vi "AK Befehl Auswerten - PEUS.vi"(10 "Array":string[](array[string])) -> (2 "String für schreiben":string)   [LabVIEW 2020, in "AK-Schnittstelle.lvlib"]
uses:
  AK-Schnittstelle.lvlib
  Aktionen Stoernummern pruefen.ctl
  Aktionen Zustandsfehlerinformation.ctl
  Aktionen Gespeicherte Werte.ctl
  Funktionstasten/Zustaende.ctl
  Funktionstasten/Funktionstasten-Aktion.ctl
  Funktionstasten/Betriebsart.ctl
  Seiten/Log Konfig/Aktionen Trigger.ctl
  Seiten/Erweiterte Konfig/FGV PID Aktionen.ctl
  Seiten/FT-IR/FGV FT-IR Diagnose Aktionen.ctl
  AK Namen Aktionen.ctl
  Seiten/System Einstellungen V2/Aktioen FGV System.ctl
  Messdaten/Aktionen FGV Messdaten.ctl
  Schedule Modul/Aktion FGV Scheduler Status.ctl
  Funktionstasten/Funktionstasten.lvlib
  Seiten/Log Konfig/LogKonfig.lvlib
  Seiten/FT-IR/FT-IR.lvlib
  Seiten/FT-IR/FGV FT-IR Gasliste Aktionen.ctl
  Messdaten/Messdaten.lvlib
  Seiten/Erweiterte Konfig/Erweiterte Konfig.lvlib
  cRIO/PC/Kommunikation mit cRIO.lvlib
  Seiten/System Einstellungen V2/System Einstellungen V2.lvlib
  Schedule Modul/Schedule Modul.lvlib
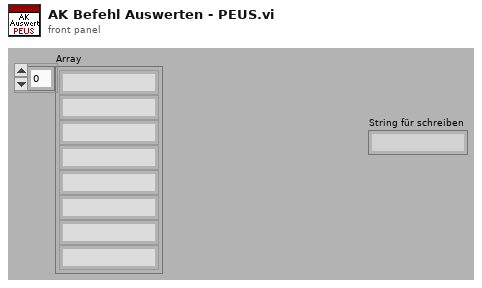
[diagram p1: front panel]
types:
  T1 = typedef "AK-Schnittstelle.lvlib/Aktionen Stoernummern pruefen.ctl" = enum16{"lesen", "prüfen"}
  T2 = typedef "AK-Schnittstelle.lvlib/Aktionen Zustandsfehlerinformation.ctl" = enum16{"OK", "Offline", "Busy", "Syntax Error", "Datenfehler"}
  T3 = typedef "AK-Schnittstelle.lvlib/Aktionen Gespeicherte Werte.ctl" = enum16{"lesen", "laden", "speichern", "Seriell", "TCP", "Diverse", "AKTIV", "AK-Namen"}
  T4 = typedef "Funktionstasten.lvlib/Zustaende.ctl" = enum16{"Standby", "Pause", "Eco", "Messen", "Kalibrieren", "Spülen Filter", "Spülen Leitung", "Umgebungsluft", "0-Gas", "Cal-Gas", "CG zu PNS", "-------------", "Init 1", "Init 2", "Init 3", "Init 4", "Messen vorbereiten", "Messen durchführen", "Exit"}
  T5 = typedef "Funktionstasten.lvlib/Betriebsart.ctl" = enum16{"Manuell", "Remote", "Bitparallel"}
  T6 = typedef "Funktionstasten.lvlib/Funktionstasten-Aktion.ctl" = enum16{"Initialisieren", "Zustand setzen", "Taste gedrückt", "Fehler speichern", "Lesen", "Manuell", "Remote", "Bitparallel", "Samplepoint", "Zeit Prüfen", "reset Umschalten"}
  T7 = typedef "LogKonfig.lvlib/Aktionen Trigger.ctl" = enum16{"lesen", "ALLE schreiben", "Trigger prüfen", "Trigger rücksetzen"}
  T8 = typedef "Erweiterte Konfig.lvlib/FGV PID Aktionen.ctl" = enum16{"Lesen", "Schreiben PID", "Schreiben Sonstige", "Dichtheitstest", "Aktionen Dicht.", "Parameter Sensor"}
  T9 = typedef "FT-IR.lvlib/FGV FT-IR Diagnose Aktionen.ctl" = enum16{"Lesen", "Diagnose Schreiben", "Min Schreiben", "Max Schreiben"}
  T10 = typedef "AK-Schnittstelle.lvlib/AK Namen Aktionen.ctl" = enum16{"lesen", "laden", "speichern Namen", "AK Namen", "Liste erstellen", "EKFG erstellen", "speichern EKFG", "EKFG schreiben", "Neuen Eintrag erzeugen"}
  T11 = typedef "FT-IR.lvlib/FGV FT-IR Gasliste Aktionen.ctl" = enum16{"lesen", "Gasliste FT-IR", "Gasliste ausgelesen", "laden", "speichern", "löschen"}
  T12 = typedef "System Einstellungen V2.lvlib/Aktioen FGV System.ctl" = enum16{"lesen", "laden", "speichern", "Optionen schreiben", "Zeitstempel", "Reset BMP", "Reset SQP", "Wartung", "Werkseinstellung"}
  T13 = typedef "Messdaten.lvlib/Aktionen FGV Messdaten.ctl" = enum16{"lesen", "schreiben", "löschen", "Mittelwerte", "Komponente"}
  T14 = typedef "Schedule Modul.lvlib/Aktion FGV Scheduler Status.ctl" = enum16{"lesen", "init", "aktiv", "inaktiv"}
  T15 = typedef "AK-Schnittstelle.lvlib/Diverse gespeicherte Werte.ctl" = cluster{"Kalibriergaseingang":i16, "SamplePoint":i16, "CalGas zu PNS":i16, "Gas-Reihenfolge":i16[], "Zeit 0-Gas":sgl, "Zeit CalGas":sgl, "AK Befehlssatz":T16}
  T16 = typedef "AK-Schnittstelle.lvlib/AK Befehlssatz.ctl" = enum16{"MEXA", "IAG v1.4", "AVL (Puma)", "PEUS"}
  T17 = typedef "LogKonfig.lvlib/Element Triggerereignisse.ctl" = cluster{"Trigger verwenden":T18, "Messwert":u16, "kl./gr.":u16, "Wert":sgl, "Puffergröße":sgl}
  T18 = typedef "LogKonfig.lvlib/Auswahlfeld aktiviert-deaktiviert.ctl" = u16
  T19 = typedef "Verwaltung - cRIO.lvlib/Analog Eingaenge.ctl" = cluster{"AI0: Durchfluss FT-IR":sgl, "AI1: Druck Ausgang":sgl, "AI2: Umgebungsdruck":sgl, "AI3: Druck FT-IR":sgl, "AI4: Druck CalGas":sgl, "AI5: Reserve":sgl, "AI6: Reserve":sgl, "AI7: Reserve":sgl, "Rohwert Durchfluss FT-IR":sgl, "Rohwert Druck Ausgang":sgl, "Rohwert Umgebungsdruck":sgl, "Rohwert Druck FT-IR":sgl, "Rohwert Druck CalGas":sgl, "Rohwert AI5":sgl, "Rohwert AI6":sgl, "Rohwert AI7":sgl, "Rohwert Diffdruck mbar FTIR":sgl}
  T20 = typedef "System Einstellungen V2.lvlib/Optionen.ctl" = cluster{"Störmeldep.":bool, "Betriebszustände":bool, "AK in ppm":bool, "log Cal-Gas":bool, "log 0-Gas":bool, "Durchflusssensor 0-5V":bool, "PNS?":bool, "Mit N2 spülen":bool, "TRE08":bool, "Amium 10-Fach":bool, "Verticale Scrollbar aktiv":bool, "Loggingtakt":bool, "AK Rezeptwechsel gleich wie MKS":bool, "NG ECO":bool}
  T21 = typedef "Verwaltung - cRIO.lvlib/TC Eingaenge.ctl" = cluster{"TC0: Reserve":sgl, "TC1: HL zu FT-IR":sgl, "TC2: HL Extern SP1":sgl, "TC3: HL Extern SP2":sgl, "TC4: Reserve":sgl, "TC5: Reserve":sgl, "TC6: Reserve":sgl, "TC7: Reserve":sgl, "TC8: FT-IR":sgl, "TC9: Reserve":sgl, "TC10: Schaltschrank":sgl, "TC11: Umgebung":sgl}
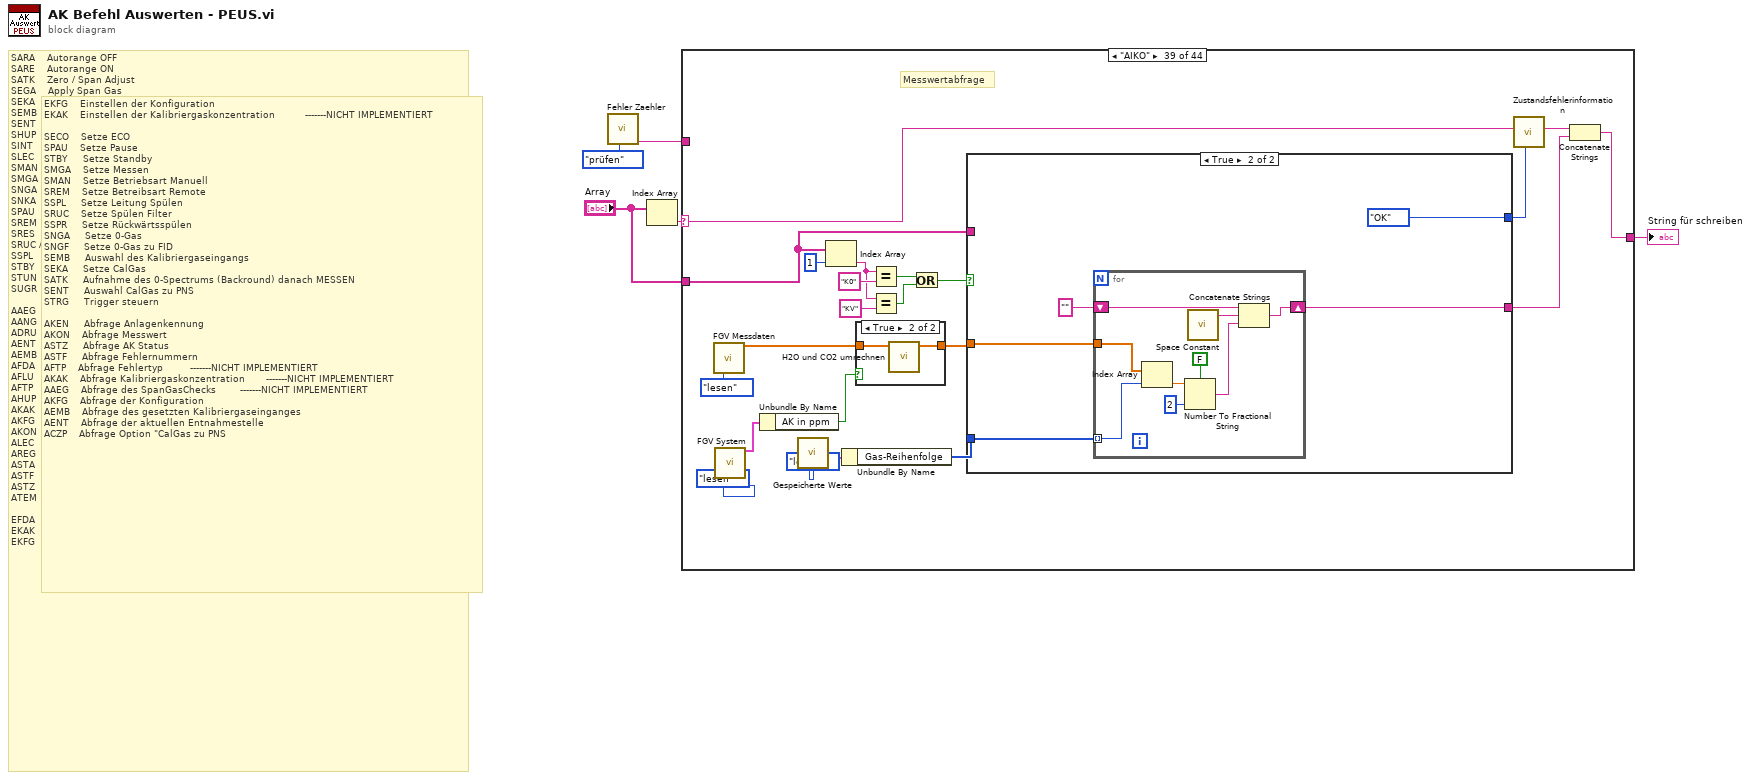
[diagram p0: block diagram]
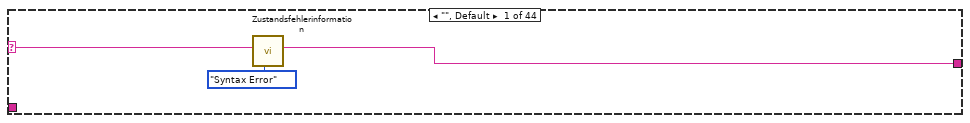
[diagram p2: hidden frame]
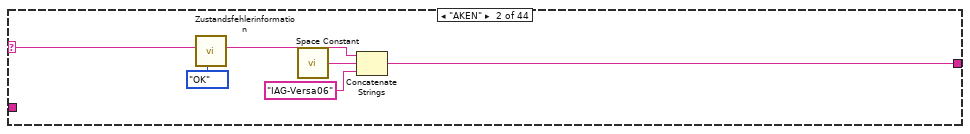
[diagram p3: hidden frame]
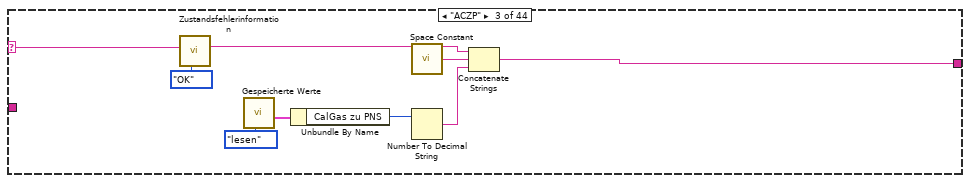
[diagram p4: hidden frame]
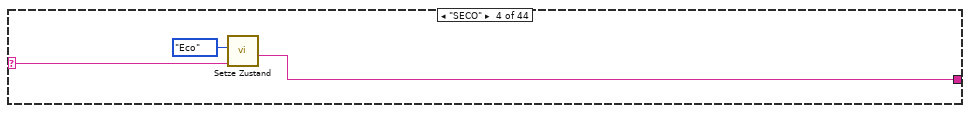
[diagram p5: hidden frame]
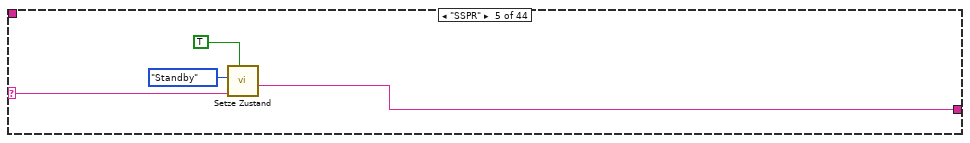
[diagram p6: hidden frame]
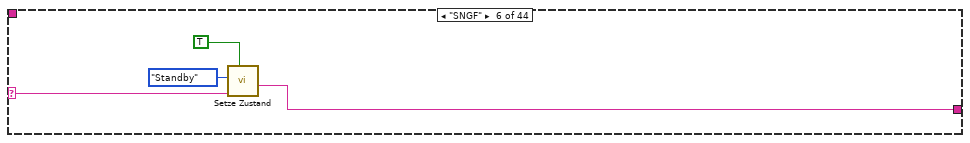
[diagram p7: hidden frame]
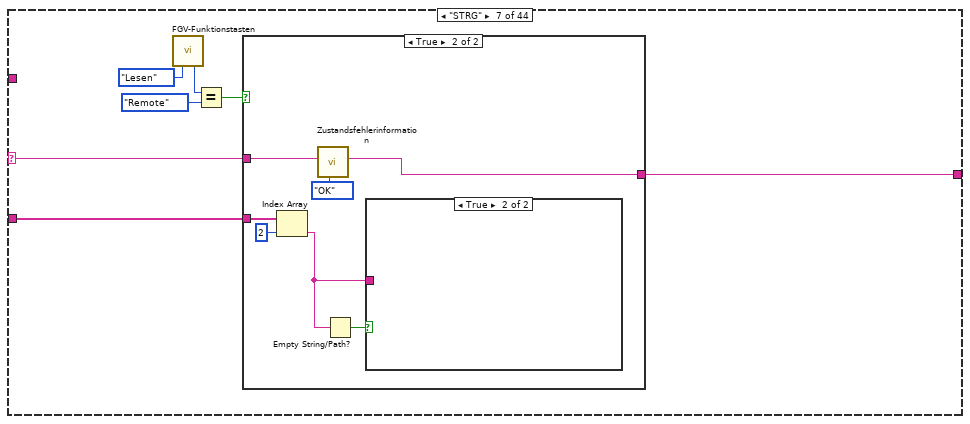
[diagram p8: hidden frame]
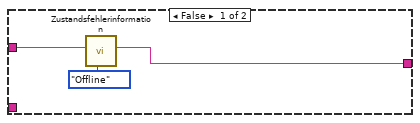
[diagram p9: hidden frame]
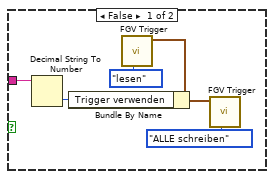
[diagram p10: hidden frame]
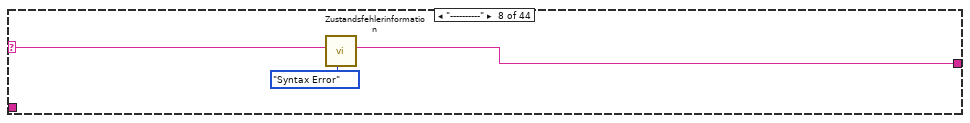
[diagram p11: hidden frame]
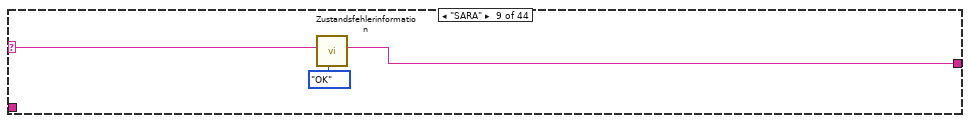
[diagram p12: hidden frame]
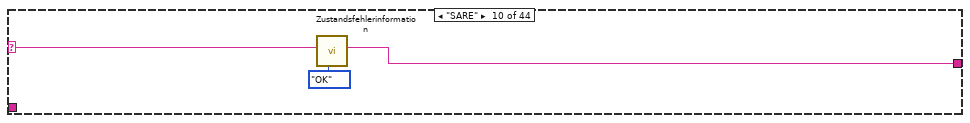
[diagram p13: hidden frame]
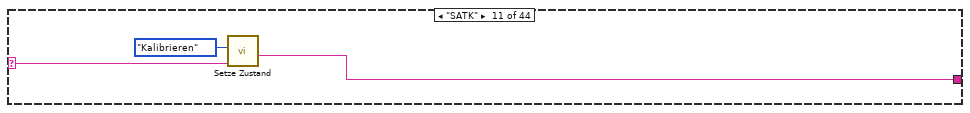
[diagram p14: hidden frame]
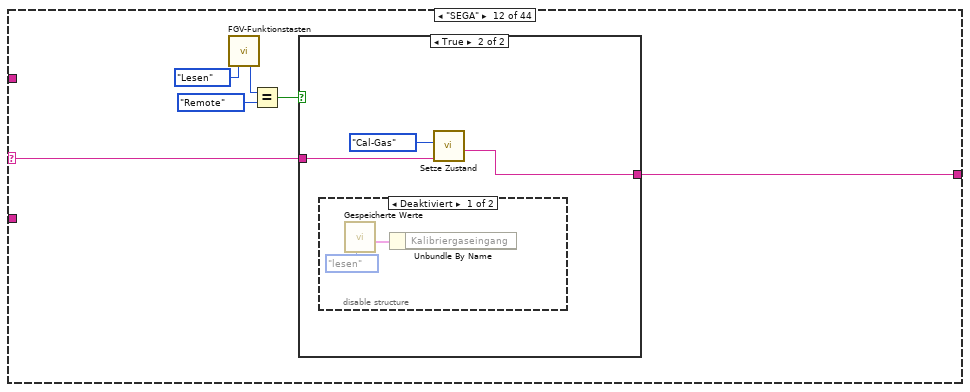
[diagram p15: hidden frame]
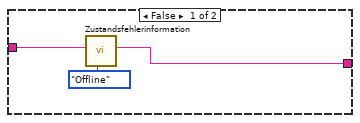
[diagram p16: hidden frame]
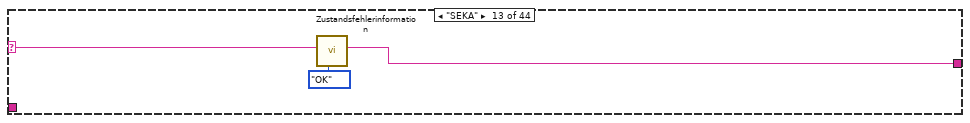
[diagram p18: hidden frame]
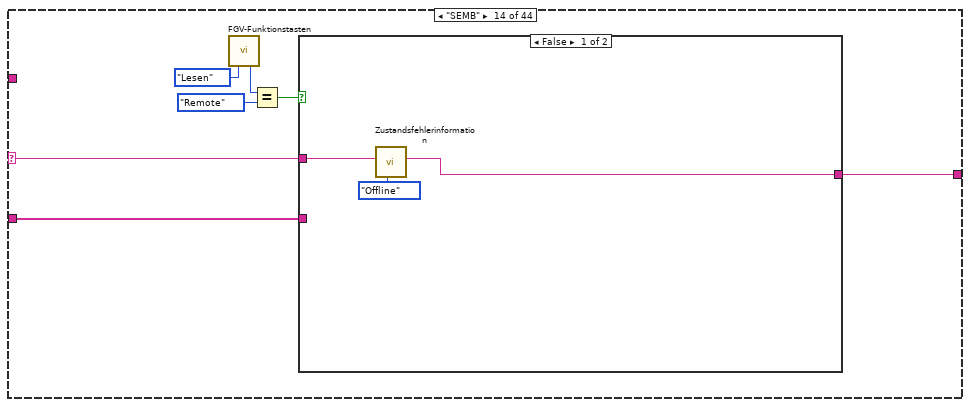
[diagram p19: hidden frame]
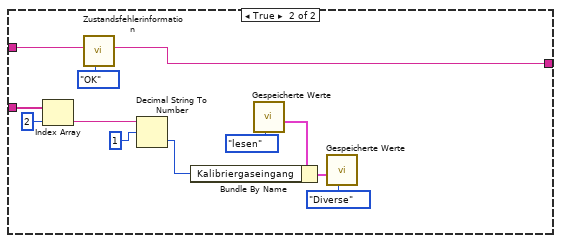
[diagram p20: hidden frame]
diagram:
  # "SARA    Autorange OFF\nSARE    Autorange ON\nSATK    Zero / Span Adjust\nSEGA    Apply Span Gas\nSEKA    Performing FTIR Span Gas Check\nSEMB    Selecting Calibration Gas Inlet\nSENT    Set Sampling\nSHUP    Hang-Up Test         -------NICHT IMPLEMENTIERT\nSINT     Starting Continous FTIR Measurement\nSLEC     Leak Check\nSMAN    Set Manual\nSMGA    Set Measure\nSNGA    Apply Zero Gas\nSNKA    Adjust Zero Point\nSPAU    Pause Modus\nSREM    Set Remote\nSRES    Set Reset\nSRUC / SRUK  Backflush\nSSPL     Purge Gas Lines\nSTBY    Set Standby\nSTUN    Automatically Adjusting Optics and Signals         -------NICHT IMPLEMENTIERT\nSUGR    Recording Zero Energy Spectrum\n\nAAEG    Inquire Span Point Deviation\nAANG    Inquire Zero Point Deviation\nADRU    Inquire Pressure of SESAM FTIR\nAENT    Inquire Sampling Points\nAEMB    Inquire Measuring Range\nAFDA    Inquire Function Duration\nAFLU     Inquire Sample Flow of SBEAM FTIR\nAFTP     Inquire Error Type\nAHUP    Inquire Hangup Result         -------NICHT IMPLEMENTIERT\nAKAK    Inquire Span Gas Concentrations         -------NICHT IMPLEMENTIERT\nAKFG    Inquire Configuration\nAKON   Inquire Measuring Value\nALEC    Inquire Leak Check Result         -------NICHT IMPLEMENTIERT\nAREG    Inquire Control Variable of SESAM FTIR          -------NICHT IMPLEMENTIERT\nASTA    Inquire Erroneous Channel         -------NICHT IMPLEMENTIERT\nASTF    Inquire Error Numbers\nASTZ    Inquire AK Status\nATEM   Inquire Temperature of SESAM FTIR\n\nEFDA   Configure Function Duration\nEKAK   Configure Span Gas Concentration         -------NICHT IMPLEMENTIERT\nEKFG   Configure Configuration"
  # "EKFG    Einstellen der Konfiguration\nEKAK    Einstellen der Kalibriergaskonzentration          -------NICHT IMPLEMENTIERT\n\nSECO    Setze ECO\nSPAU    Setze Pause\nSTBY     Setze Standby\nSMGA    Setze Messen\nSMAN    Setze Betriebsart Manuell\nSREM    Setze Betreibsart Remote\nSSPL     Setze Leitung Spülen\nSRUC    Setze Spülen Filter\nSSPR     Setze Rückwärtsspülen\nSNGA     Setze 0-Gas\nSNGF     Setze 0-Gas zu FID\nSEMB     Auswahl des Kalibriergaseingangs\nSEKA     Setze CalGas\nSATK     Aufnahme des 0-Spectrums (Backround) danach MESSEN\nSENT     Auswahl CalGas zu PNS\nSTRG     Trigger steuern\n\nAKEN     Abfrage Anlagenkennung\nAKON    Abfrage Messwert\nASTZ     Abfrage AK Status\nASTF     Abfrage Fehlernummern\nAFTP    Abfrage Fehlertyp         -------NICHT IMPLEMENTIERT\nAKAK    Abfrage Kalibriergaskonzentration       -------NICHT IMPLEMENTIERT\nAAEG    Abfrage des SpanGasChecks        -------NICHT IMPLEMENTIERT\nAKFG    Abfrage der Konfiguration\nAEMB    Abfrage des gesetzten Kalibriergaseinganges\nAENT    Abfrage der aktuellen Entnahmestelle\nACZP    Abfrage Option \"CalGas zu PNS"
  n1 = call "Fehler Zaehler.vi"("Aktionen"=Aktionen_Stoernummern_pruefen."prüfen") -> ("Fehlerzähler"=w3:string)  [unwired: 7 in, 3 out]
  n2 = Index Array(array="Array") -> (element=w2:string)  [unwired: 1 in]
  n3 = case shown="\"AIKO\"" w2 {
    selector: w2 -> [w7 w11 w21 w26 w30 w34 w37 w59 w62 w65 w68 w71 w85 w89 w112 w149 w152 w162 w176 w179 w181 w185 w187 w191 w195 w198 w201 w204 w206 w220 w228 w244 w250 w256 w287 w297 w305 w365 w439 w493 w511 w563 w572 w600]
    tunnel: [w6 w13 w23 w25 w29 w33 w36 w58 w61 w64 w67 w70 w84 w88 w111 w148 w151 w161 w175 w178 w180 w184 w186 w190 w194 w197 w200 w203 w205 w222 w230 w246 w252 w257 w289 w299 w307 w366 w440 w495 w509 w565 w571 w599] -> w5
    tunnel: w3 -> [_ _ _ _ _ _ _ _ _ _ _ _ _ _ _ _ _ _ _ _ _ _ _ _ _ _ _ _ _ _ _ _ _ _ _ _ _ _ _ _ _ _ _ _]
    tunnel: "Array" -> [_ _ _ _ _ _ w35 _ _ _ _ _ _ w87 w110 _ _ _ _ _ _ _ _ _ _ _ _ _ _ _ _ _ _ w255 _ _ w302 w359 w433 _ w510 _ w570 w601]
    frame "", Default {
      n4 = call "Zustandsfehlerinformation.vi"("Aktionen"=Aktionen_Zustandsfehlerinformation."Syntax Error", "String"=w7) -> ("String"=w6:string)  [unwired: 9 in]
    }
    frame "AKEN" {
      n5 = call "Zustandsfehlerinformation.vi"("Aktionen"=Aktionen_Zustandsfehlerinformation."OK", "String"=w11) -> ("String"=w10:string)  [unwired: 9 in]
      n6 = call <vilib>:"Space Constant.vi"() -> ("String"=w9:string)
      n7 = Concatenate Strings(w10, w9, "IAG-Versa06" ("String")) -> (w13:string)
    }
    frame "ACZP" {
      n8 = call "Zustandsfehlerinformation.vi"("Aktionen"=Aktionen_Zustandsfehlerinformation."OK", "String"=w21) -> ("String"=w20:string)  [unwired: 9 in]
      n9 = call "Gespeicherte Werte.vi"("Aktionen"=Aktionen_Gespeicherte_Werte."lesen") -> ("Diverse Werte"=w15:T15)  [unwired: 6 in, 4 out]
      n10 = Unbundle By Name(w15) -> ("CalGas zu PNS"=w18:i16)
      n11 = call <vilib>:"Space Constant.vi"() -> ("String"=w16:string)
      n12 = Number To Decimal String(number=w18) -> (decimal integer string=w17:string)  [unwired: 1 in]
      n13 = Concatenate Strings(w20, w16, w17) -> (w23:string)
    }
    frame "SECO" {
      n14 = call "Setze Zustand.vi"("AK Befehl"=w26, "Zustand"=Zustaende."Eco") -> ("Antwort String"=w25:string)  [unwired: 8 in, 1 out]
    }
    frame "SSPR" {
      n15 = call "Setze Zustand.vi"("Befehl nicht vorhanden!"=TRUE, "AK Befehl"=w30, "Zustand"=Zustaende."Standby") -> ("Antwort String"=w29:string)  [unwired: 7 in, 1 out]
    }
    frame "SNGF" {
      n16 = call "Setze Zustand.vi"("Befehl nicht vorhanden!"=TRUE, "AK Befehl"=w34, "Zustand"=Zustaende."Standby") -> ("Antwort String"=w33:string)  [unwired: 7 in, 1 out]
    }
    frame "STRG" {
      n17 = call "FGV-Funktionstasten.vi"("Aktion"=Funktionstasten-Aktion."Lesen") -> ("Betriebsart"=w40:T5)  [unwired: 7 in, 7 out]
      n18 = Equal?(x=w40, y=Betriebsart."Remote" ("Betriebsart")) -> (x = y?=w41:bool)
      n19 = case shown="True" w41 {
        tunnel: w37 -> [w43 w50]
        tunnel: [w42 w49] -> w36
        tunnel: w35 -> [_ w48]
        frame False {
          n20 = call "Zustandsfehlerinformation.vi"("Aktionen"=Aktionen_Zustandsfehlerinformation."Offline", "String"=w43) -> ("String"=w42:string)  [unwired: 9 in]
        }
        frame True {
          n21 = Index Array(array=w48, index=2 ("Index")) -> (element=w46:string)
          n22 = call "Zustandsfehlerinformation.vi"("Aktionen"=Aktionen_Zustandsfehlerinformation."OK", "String"=w50) -> ("String"=w49:string)  [unwired: 9 in]
          n23 = Empty String/Path?(string/path=w46) -> (empty?=w45:bool)
          n24 = case shown="True" w45 {
            tunnel: w46 -> [w57 _]
            frame False {
              n25 = Decimal String To Number(string=w57) -> (number=w54:i32)  [unwired: 2 in, 1 out]
              n26 = call "FGV Trigger.vi"("Aktion"=Aktionen_Trigger."lesen") -> ("Triggerereignis neu"=w53:T17)  [unwired: 7 in, 3 out]
              n27 = Bundle By Name(cluster=w53, "Trigger verwenden"=w54) -> (w52:T17)
              n28 = call "FGV Trigger.vi"("Aktion"=Aktionen_Trigger."ALLE schreiben", "Triggerereignis"=w52) -> ()  [unwired: 6 in, 4 out]
            }
            frame True {
            }
          }
        }
      }
    }
    frame "----------" {
      n29 = call "Zustandsfehlerinformation.vi"("Aktionen"=Aktionen_Zustandsfehlerinformation."Syntax Error", "String"=w59) -> ("String"=w58:string)  [unwired: 9 in]
    }
    frame "SARA" {
      n30 = call "Zustandsfehlerinformation.vi"("Aktionen"=Aktionen_Zustandsfehlerinformation."OK", "String"=w62) -> ("String"=w61:string)  [unwired: 9 in]
    }
    frame "SARE" {
      n31 = call "Zustandsfehlerinformation.vi"("Aktionen"=Aktionen_Zustandsfehlerinformation."OK", "String"=w65) -> ("String"=w64:string)  [unwired: 9 in]
    }
    frame "SATK" {
      n32 = call "Setze Zustand.vi"("AK Befehl"=w68, "Zustand"=Zustaende."Kalibrieren") -> ("Antwort String"=w67:string)  [unwired: 8 in, 1 out]
    }
    frame "SEGA" {
      n33 = call "FGV-Funktionstasten.vi"("Aktion"=Funktionstasten-Aktion."Lesen") -> ("Betriebsart"=w74:T5)  [unwired: 7 in, 7 out]
      n34 = Equal?(x=w74, y=Betriebsart."Remote" ("Betriebsart")) -> (x = y?=w75:bool)
      n35 = case shown="True" w75 {
        tunnel: w71 -> [w77 w80]
        tunnel: [w76 w79] -> w70
        frame False {
          n36 = call "Zustandsfehlerinformation.vi"("Aktionen"=Aktionen_Zustandsfehlerinformation."Offline", "String"=w77) -> ("String"=w76:string)  [unwired: 9 in]
        }
        frame True {
          n37 = disable-structure shown="Deaktiviert" {
            frame Disabled {
              n38 = call "Gespeicherte Werte.vi"("Aktionen"=Aktionen_Gespeicherte_Werte."lesen") -> ("Diverse Werte"=w82:T15)  [unwired: 6 in, 4 out]
              n39 = Unbundle By Name(w82) -> ()  [unwired: 1 out]
            }
            frame Enabled {
            }
          }
          n40 = call "Setze Zustand.vi"("AK Befehl"=w80, "Zustand"=Zustaende."Cal-Gas") -> ("Antwort String"=w79:string)  [unwired: 8 in, 1 out]
        }
      }
    }
    frame "SEKA" {
      n41 = call "Zustandsfehlerinformation.vi"("Aktionen"=Aktionen_Zustandsfehlerinformation."OK", "String"=w85) -> ("String"=w84:string)  [unwired: 9 in]
    }
    frame "SEMB" {
      n42 = call "FGV-Funktionstasten.vi"("Aktion"=Funktionstasten-Aktion."Lesen") -> ("Betriebsart"=w92:T5)  [unwired: 7 in, 7 out]
      n43 = Equal?(x=w92, y=Betriebsart."Remote" ("Betriebsart")) -> (x = y?=w93:bool)
      n44 = case shown="False" w93 {
        tunnel: w89 -> [w95 w107]
        tunnel: [w94 w106] -> w88
        tunnel: w87 -> [_ w105]
        frame False {
          n45 = call "Zustandsfehlerinformation.vi"("Aktionen"=Aktionen_Zustandsfehlerinformation."Offline", "String"=w95) -> ("String"=w94:string)  [unwired: 9 in]
        }
        frame True {
          n46 = Index Array(array=w105, index=2 ("Index")) -> (element=w98:string)
          n47 = call "Zustandsfehlerinformation.vi"("Aktionen"=Aktionen_Zustandsfehlerinformation."OK", "String"=w107) -> ("String"=w106:string)  [unwired: 9 in]
          n48 = Decimal String To Number(string=w98, offset=1 ("Offset (0)")) -> (number=w97:i32)  [unwired: 1 in, 1 out]
          n49 = call "Gespeicherte Werte.vi"("Aktionen"=Aktionen_Gespeicherte_Werte."lesen") -> ("Diverse Werte"=w100:T15)  [unwired: 6 in, 4 out]
          n50 = Bundle By Name(cluster=w100, "Kalibriergaseingang"=w97) -> (w99:T15)
          n51 = call "Gespeicherte Werte.vi"("Aktionen"=Aktionen_Gespeicherte_Werte."Diverse", "Diverse Werte"=w99) -> ()  [unwired: 5 in, 5 out]
        }
      }
    }
    frame "SENT" {
      n52 = call "FGV-Funktionstasten.vi"("Aktion"=Funktionstasten-Aktion."Lesen") -> ("Betriebsart"=w115:T5)  [unwired: 7 in, 7 out]
      n53 = Equal?(x=w115, y=Betriebsart."Remote" ("Betriebsart")) -> (x = y?=w109:bool)
      n54 = case shown="True" w109 {
        tunnel: w112 -> [w117 w131]
        tunnel: [w116 w130] -> w111
        tunnel: w110 -> [_ w120]
        frame False {
          n55 = call "Zustandsfehlerinformation.vi"("Aktionen"=Aktionen_Zustandsfehlerinformation."Offline", "String"=w117) -> ("String"=w116:string)  [unwired: 9 in]
        }
        frame True {
          n56 = Index Array(array=w120, index=2 ("Index")) -> (element=w122:string)
          n57 = Equal?(x=w122, y="L1") -> (x = y?=w119:bool)
          n58 = case shown="True" w119 {
            tunnel: [w142 w143] -> w124
            tunnel: w120 -> [w133 w145]
            frame False {
              n59 = Array Size(array=w133) -> (size(s)=w140:i32)
              n60 = Greater?(x=w140, y=3) -> (0:w138:bool)
              n61 = Select(t=3, s=w138, f=2 ("Index")) -> (s? t:f=w135:i32)
              n62 = Index Array(array=w133, index=w135) -> (element=w134:string)
              n63 = Decimal String To Number(string=w134, offset=1 ("Offset")) -> (number=w142:i32)  [unwired: 1 in, 1 out]
            }
            frame True {
              n64 = Index Array(array=w145, index=3 ("Index")) -> (element=w144:string)
              n65 = Decimal String To Number(string=w144) -> (number=w143:i32)  [unwired: 2 in, 1 out]
            }
          }
          n66 = call "FGV-Funktionstasten.vi"("Samplepoint"=w124, "Aktion"=Funktionstasten-Aktion."Samplepoint") -> ()  [unwired: 6 in, 8 out]
          n67 = call "Zustandsfehlerinformation.vi"("Aktionen"=Aktionen_Zustandsfehlerinformation."OK", "String"=w131) -> ("String"=w130:string)  [unwired: 9 in]
          n68 = call "Gespeicherte Werte.vi"("Aktionen"=Aktionen_Gespeicherte_Werte."lesen") -> ("Diverse Werte"=w127:T15)  [unwired: 6 in, 4 out]
          n69 = Bundle By Name(cluster=w127, "SamplePoint"=w124) -> (w126:T15)
          n70 = call "Gespeicherte Werte.vi"("Aktionen"=Aktionen_Gespeicherte_Werte."Diverse", "Diverse Werte"=w126) -> ()  [unwired: 5 in, 5 out]
        }
      }
    }
    frame "SINT" {
      n71 = call "Setze Zustand.vi"("AK Befehl"=w149, "Zustand"=Zustaende."Messen") -> ("Antwort String"=w148:string)  [unwired: 8 in, 1 out]
    }
    frame "SLEC" {
      n72 = flat-sequence {
        frame #0 {
          n73 = call "FGV Erweiterte Konfig.vi"("Aktion"=FGV_PID_Aktionen."Dichtheitstest", "Dichtheitstest?"=TRUE) -> ()  [unwired: 5 in, 5 out]
        }
        frame #1 {
          n74 = vi-ref "Dichtheitstest.vi"() -> (w157:refnum<vi>)
          n75 = invoke class="VI" method="VI ausführen"(reference=w157, "Wait until done"=FALSE ("Warten bis beendet"), "Auto Dispose Ref"=TRUE ("Referenz automatisch schließen")) -> (reference out=w158:refnum<vi>, error out=w156:errorcluster)  [unwired: 2 in, 3 out]
          n76 = invoke class="VI" method="FP.Öffnen"(reference=w158, error in=w156) -> (error out=w155:errorcluster)  [unwired: 3 in, 4 out]
          n77 = call <vilib>:"Clear Errors.vi"("error in (no error)"=w155) -> ()  [unwired: 5 in, 2 out]
        }
      }
      n78 = call "Setze Zustand.vi"("AK Befehl"=w152, "Zustand"=Zustaende."Standby") -> ("Antwort String"=w151:string)  [unwired: 8 in, 1 out]
    }
    frame "SMAN" {
      n79 = call "FGV-Funktionstasten.vi"("Aktion"=Funktionstasten-Aktion."Lesen") -> ("Betriebsart"=w166:T5)  [unwired: 7 in, 7 out]
      n80 = Equal?(x=w166, y=Betriebsart."Remote" ("Betriebsart")) -> (x = y?=w163:bool)
      n81 = case shown="True" w163 {
        tunnel: w162 -> [w169 w172]
        tunnel: [w167 w171] -> w161
        frame False {
          n82 = call "Zustandsfehlerinformation.vi"("Aktionen"=Aktionen_Zustandsfehlerinformation."Offline", "String"=w169) -> ("String"=w167:string)  [unwired: 9 in]
        }
        frame True {
          n83 = call "Zustandsfehlerinformation.vi"("Aktionen"=Aktionen_Zustandsfehlerinformation."OK", "String"=w172) -> ("String"=w171:string)  [unwired: 9 in]
          n84 = call "FGV-Funktionstasten.vi"("Aktion"=Funktionstasten-Aktion."Manuell") -> ()  [unwired: 7 in, 8 out]
        }
      }
    }
    frame "SMGA" {
      n85 = call "Setze Zustand.vi"("AK Befehl"=w176, "Zustand"=Zustaende."Messen") -> ("Antwort String"=w175:string)  [unwired: 8 in, 1 out]
    }
    frame "SNGA" {
      n86 = call "Setze Zustand.vi"("AK Befehl"=w179, "Zustand"=Zustaende."0-Gas") -> ("Antwort String"=w178:string)  [unwired: 8 in, 1 out]
    }
    frame "SNKA" {
      n87 = call "Zustandsfehlerinformation.vi"("Aktionen"=Aktionen_Zustandsfehlerinformation."OK", "String"=w181) -> ("String"=w180:string)  [unwired: 9 in]
    }
    frame "SPAU" {
      n88 = call "Setze Zustand.vi"("AK Befehl"=w185, "Zustand"=Zustaende."Pause") -> ("Antwort String"=w184:string)  [unwired: 8 in, 1 out]
    }
    frame "SREM" {
      n89 = call "Zustandsfehlerinformation.vi"("Aktionen"=Aktionen_Zustandsfehlerinformation."OK", "String"=w187) -> ("String"=w186:string)  [unwired: 9 in]
      n90 = call "FGV-Funktionstasten.vi"("Aktion"=Funktionstasten-Aktion."Remote") -> ()  [unwired: 7 in, 8 out]
    }
    frame "SRES" {
      n91 = call "Zustandsfehlerinformation.vi"("Aktionen"=Aktionen_Zustandsfehlerinformation."OK", "String"=w191) -> ("String"=w190:string)  [unwired: 9 in]
    }
    frame "SRUC" {
      n92 = call "Setze Zustand.vi"("AK Befehl"=w195, "Zustand"=Zustaende."Spülen Filter") -> ("Antwort String"=w194:string)  [unwired: 8 in, 1 out]
    }
    frame "SRUK" {
      n93 = call "Setze Zustand.vi"("AK Befehl"=w198, "Zustand"=Zustaende."Spülen Filter") -> ("Antwort String"=w197:string)  [unwired: 8 in, 1 out]
    }
    frame "SSPL" {
      n94 = call "Setze Zustand.vi"("AK Befehl"=w201, "Zustand"=Zustaende."Spülen Leitung") -> ("Antwort String"=w200:string)  [unwired: 8 in, 1 out]
    }
    frame "STBY" {
      n95 = call "Setze Zustand.vi"("AK Befehl"=w204, "Zustand"=Zustaende."Standby") -> ("Antwort String"=w203:string)  [unwired: 8 in, 1 out]
    }
    frame "SUGR" {
      n96 = call "Setze Zustand.vi"("AK Befehl"=w206, "Zustand"=Zustaende."Kalibrieren") -> ("Antwort String"=w205:string)  [unwired: 8 in, 1 out]
    }
    frame "ADRU" {
      w209 = "00.0" ("String in F-Format")
      n97 = call "Zustandsfehlerinformation.vi"("Aktionen"=Aktionen_Zustandsfehlerinformation."OK", "String"=w220) -> ("String"=w219:string)  [unwired: 9 in]
      n98 = call "FGV FT-IR Diagnosewerte.vi"("Aktionen"=FGV_FT-IR_Diagnose_Aktionen."Lesen") -> ("Druck"=w216:dbl)  [unwired: 5 in, 5 out]
      n99 = Multiply(x=w216, y=1000.0) -> (x*y=w213:dbl)
      n100 = call <vilib>:"Space Constant.vi"() -> ("String"=w210:string)
      n101 = Number To Fractional String(use system decimal point (T)=FALSE ("Systemdezimalzeichen verwenden (T)"), number=w213, precision (6)=i16 1 ("Genauigkeit (6)")) -> (F-format string=w211:string)  [unwired: 1 in]
      n102 = Concatenate Strings(w210, w209, w210, w209, w210, w209) -> (w208:string)
      n103 = call <vilib>:"Space Constant.vi"() -> ("String"=w218:string)
      n104 = Concatenate Strings(w219, w218, w211, w208) -> (w222:string)
    }
    frame "AENT" {
      n105 = call "Zustandsfehlerinformation.vi"("Aktionen"=Aktionen_Zustandsfehlerinformation."OK", "String"=w228) -> ("String"=w227:string)  [unwired: 9 in]
      n106 = call "FGV-Funktionstasten.vi"("Aktion"=Funktionstasten-Aktion."Lesen") -> ("Samplepoint"=w224:u16)  [unwired: 7 in, 7 out]
      n107 = call <vilib>:"Space Constant.vi"() -> ("String"=w226:string)
      n108 = Number To Decimal String(number=w224) -> (decimal integer string=w223:string)  [unwired: 1 in]
      n109 = Concatenate Strings(w227, w226, w223) -> (w230:string)
      n110 = disable-structure shown="Deaktiviert" {
        frame Disabled {
          n111 = call "FGV-Funktionstasten.vi"("Aktion"=Funktionstasten-Aktion."Lesen") -> ("Samplepoint"=w231:u16)  [unwired: 7 in, 7 out]
          n112 = call <vilib>:"Space Constant.vi"() -> ("String"=w233:string)
          n113 = Number To Decimal String(number=w231) -> (decimal integer string=w234:string)  [unwired: 1 in]
          n114 = Concatenate Strings(w233, "M" ("String"), w234) -> (w236:string)  [unwired: 1 out]
        }
        frame Enabled {
        }
      }
    }
    frame "AEMB" {
      n115 = call "Zustandsfehlerinformation.vi"("Aktionen"=Aktionen_Zustandsfehlerinformation."OK", "String"=w244) -> ("String"=w243:string)  [unwired: 9 in]
      n116 = call "Gespeicherte Werte.vi"("Aktionen"=Aktionen_Gespeicherte_Werte."lesen") -> ("Diverse Werte"=w237:T15)  [unwired: 6 in, 4 out]
      n117 = Unbundle By Name(w237) -> ("Kalibriergaseingang"=w241:i16)
      n118 = call <vilib>:"Space Constant.vi"() -> ("String"=w238:string)
      n119 = Number To Decimal String(number=w241) -> (decimal integer string=w239:string)  [unwired: 1 in]
      n120 = Concatenate Strings(w243, w238, "M" ("String"), w239) -> (w246:string)
    }
    frame "ASTA" {
      n121 = call "Zustandsfehlerinformation.vi"("Aktionen"=Aktionen_Zustandsfehlerinformation."OK", "String"=w250) -> ("String"=w249:string)  [unwired: 9 in]
      n122 = call <vilib>:"Space Constant.vi"() -> ("String"=w247:string)
      n123 = Concatenate Strings(w249, w247, "KV" ("String")) -> (w252:string)
    }
    frame "AFDA" {
      n124 = Index Array(array=w255, index=2 ("Index")) -> (element=w253:string)
      n125 = case shown="\" \", Standard" w253 {
        tunnel: [w258 w269 w278] -> w257
        tunnel: w256 -> [w259 w267 w276]
        frame " ", Default {
          n126 = call "Zustandsfehlerinformation.vi"("Aktionen"=Aktionen_Zustandsfehlerinformation."Datenfehler", "String"=w259) -> ("String"=w258:string)  [unwired: 9 in]
        }
        frame "SNGA" {
          n127 = call "Gespeicherte Werte.vi"("Aktionen"=Aktionen_Gespeicherte_Werte."lesen") -> ("Diverse Werte"=w264:T15)  [unwired: 6 in, 4 out]
          n128 = Unbundle By Name(w264) -> ("Zeit 0-Gas"=w262:sgl)
          n129 = call "Zustandsfehlerinformation.vi"("Aktionen"=Aktionen_Zustandsfehlerinformation."OK", "String"=w267) -> ("String"=w266:string)  [unwired: 9 in]
          n130 = call <vilib>:"Space Constant.vi"() -> ("String"=w265:string)
          n131 = Number To Decimal String(number=w262) -> (decimal integer string=w261:string)  [unwired: 1 in]
          n132 = Concatenate Strings(w266, w265, w261) -> (w269:string)
        }
        frame "SEGA" {
          n133 = call "Gespeicherte Werte.vi"("Aktionen"=Aktionen_Gespeicherte_Werte."lesen") -> ("Diverse Werte"=w273:T15)  [unwired: 6 in, 4 out]
          n134 = Unbundle By Name(w273) -> ("Zeit CalGas"=w271:sgl)
          n135 = call "Zustandsfehlerinformation.vi"("Aktionen"=Aktionen_Zustandsfehlerinformation."OK", "String"=w276) -> ("String"=w275:string)  [unwired: 9 in]
          n136 = call <vilib>:"Space Constant.vi"() -> ("String"=w274:string)
          n137 = Number To Decimal String(number=w271) -> (decimal integer string=w270:string)  [unwired: 1 in]
          n138 = Concatenate Strings(w275, w274, w270) -> (w278:string)
        }
      }
    }
    frame "AFLU" {
      n139 = call "Zustandsfehlerinformation.vi"("Aktionen"=Aktionen_Zustandsfehlerinformation."OK", "String"=w287) -> ("String"=w286:string)  [unwired: 9 in]
      n140 = call "FGV cRIO-Daten.vi"("Aktion"=enum16{"lesen", "schreiben"}."lesen") -> ("Analog Input"=w283:T19)  [unwired: 9 in, 9 out]
      n141 = Unbundle By Name(w283) -> ("AI0: Durchfluss FT-IR"=w280:sgl)
      n142 = Number To Fractional String(use system decimal point (T)=FALSE ("Systemdezimalzeichen verwenden (T)"), number=w280, precision (6)=i16 1 ("Genauigkeit (6)")) -> (F-format string=w279:string)  [unwired: 1 in]
      n143 = call <vilib>:"Space Constant.vi"() -> ("String"=w285:string)
      n144 = Concatenate Strings(w286, w285, w279) -> (w289:string)
    }
    frame "AFTP" {
      # "Fehlertyp"
      # "Fehler-Anzahl"
      n145 = call "Zustandsfehlerinformation.vi"("Aktionen"=Aktionen_Zustandsfehlerinformation."OK", "String"=w297) -> ("String"=w296:string)  [unwired: 9 in]
      n146 = call "Fehler Zaehler.vi"("Aktionen"=Aktionen_Stoernummern_pruefen."lesen") -> ("Fehler Nummern"=w294:i32[])  [unwired: 7 in, 3 out]
      n147 = Array Size(array=w294) -> (size(s)=w293:i32)
      n148 = Number To Decimal String(number=w293) -> (decimal integer string=w290:string)  [unwired: 1 in]
      n149 = call <vilib>:"Space Constant.vi"() -> ("String"=w292:string)
      n150 = Concatenate Strings(w296, w292, w290, w292, "0" ("String")) -> (w299:string)
    }
    frame "AKFG" {
      n151 = Index Array(array=w302, index=1 ("Index")) -> (element=w300:string)
      n152 = disable-structure shown="Deaktiviert" {
        frame Disabled {
          n153 = call "FGV Gasliste.vi"("Aktionen"=FGV_FT-IR_Gasliste_Aktionen."lesen") -> ()  [unwired: 8 in, 3 out]
        }
        frame Enabled {
        }
      }
      n154 = case shown="\"K0\", Standard" w300 {
        tunnel: [w308 w322] -> w303
        frame "KV " {
          n155 = call "Gespeicherte Werte.vi"("Aktionen"=Aktionen_Gespeicherte_Werte."lesen") -> ("Diverse Werte"=w312:T15)  [unwired: 6 in, 4 out]
          n156 = Unbundle By Name(w312) -> ("Gas-Reihenfolge"=w310:i16[])
          n157 = for {
            tunnel: w310 -> [w315] mode=indexing
            shift-right: [w319] -> w308
            shift-left: "" -> [w318]
            n158 = Increment(x=w315) -> (x+1=w316:i16)
            n159 = Number To Decimal String(number=w316) -> (decimal integer string=w313:string)  [unwired: 1 in]
            n160 = call <vilib>:"Space Constant.vi"() -> ("String"=w317:string)
            n161 = Concatenate Strings(w318, w317, "K" ("String"), w313) -> (w319:string)
          }
        }
        frame "K0", Default {
          n162 = call "Gespeicherte Werte.vi"("Aktionen"=Aktionen_Gespeicherte_Werte."lesen") -> ("Diverse Werte"=w323:T15)  [unwired: 6 in, 4 out]
          n163 = call "AK Namen.vi"("Aktionen"=AK_Namen_Aktionen."lesen") -> ("AK Namen"=w320:string[])  [unwired: 7 in, 3 out]
          n164 = Unbundle By Name(w323) -> ("Gas-Reihenfolge"=w325:i16[])
          n165 = for {
            tunnel: w325 -> [w335] mode=indexing
            shift-right: [w338] -> w322
            shift-left: "" -> [w337]
            tunnel: w320 -> [w336]
            i -> [w328]
            n166 = Index Array(array=w336, index=w335) -> (element=w333:string)
            n167 = for {
              N: 10 -> [_]
              shift-right: [w343] -> w332
              shift-left: w333 -> [w344]
              stop <- w341 stop-if-true
              n168 = call <vilib>:"Space Constant.vi"() -> ("String"=w340:string)
              n169 = Search and Replace String(input string=w344, search string=w340, replace string="_") -> (result string=w343:string, number of replacements=w342:i32)  [unwired: 5 in, 2 out]
              n170 = Less Or Equal To 0?(x=w342) -> (x <= 0?=w341:bool)
            }
            n171 = Increment(x=w328) -> (x+1=w330:i32)
            n172 = Number To Decimal String(number=w330) -> (decimal integer string=w327:string)  [unwired: 1 in]
            n173 = call <vilib>:"Space Constant.vi"() -> ("String"=w331:string)
            n174 = Concatenate Strings(w337, w331, w332, w331, "K" ("String"), w327) -> (w338:string)
          }
        }
      }
      n175 = call "Zustandsfehlerinformation.vi"("Aktionen"=Aktionen_Zustandsfehlerinformation."OK", "String"=w305) -> ("String"=w304:string)  [unwired: 9 in]
      n176 = Concatenate Strings(w304, w303) -> (w307:string)
    }
    frame "AKON" {
      n177 = call "FGV System.vi"("Aktionen"=Aktioen_FGV_System."lesen") -> ("Optionen"=w349:T20)  [unwired: 12 in, 6 out]
      n178 = disable-structure shown="Aktiviert" {
        disable-tunnel: [w368 w370] -> w346
        frame Disabled {
          n179 = call "FGV Messdaten.vi"("Aktionen"=Aktionen_FGV_Messdaten."lesen") -> ("Aktuelle Messwerte"=w368:sgl[])  [unwired: 6 in, 8 out]
        }
        frame Enabled {
          n180 = call "Rolling Average Umschaltung Anzeige.vi"("Aktion"=enum16{"AK", "IAG Software"}."AK") -> ("Aktuelle Messwerte"=w370:sgl[])  [unwired: 9 in, 5 out]
        }
      }
      n181 = Unbundle By Name(w349) -> ("AK in ppm"=w347:bool)
      n182 = call "Gespeicherte Werte.vi"("Aktionen"=Aktionen_Gespeicherte_Werte."lesen") -> ("Diverse Werte"=w357:T15)  [unwired: 6 in, 4 out]
      n183 = Index Array(array=w359, index=1 ("Index")) -> (element=w354:string)
      n184 = Unbundle By Name(w357) -> ("Gas-Reihenfolge"=w362:i16[])
      n185 = case shown="True" w347 {
        tunnel: w346 -> [w371 w373]
        tunnel: [w371 w372] -> w348
        frame False {
        }
        frame True {
          n186 = call "H2O und CO2 umrechnen.vi"("Aktuelle Messwerte"=w373) -> ("Aktuelle Messwerte"=w372:sgl[])  [unwired: 10 in]
        }
      }
      n187 = Equal?(x=w354, y="K0") -> (x = y?=w353:bool)
      n188 = Equal?(x=w354, y="KV") -> (x = y?=w352:bool)
      n189 = Or(x=w353, y=w352) -> (x .or. y?=w351:bool)
      n190 = case shown="True" w351 {
        tunnel: w362 -> [w376 w409]
        tunnel: [w374 w407] -> w361
        tunnel: w348 -> [w375 w406]
        tunnel: w359 -> [w380 _]
        tunnel: [w378 Aktionen_Zustandsfehlerinformation."OK" ("Aktionen")] -> w358
        frame False {
          n191 = Delete From Array(array=w380, length=1 ("Länge"), index=0 ("Index")) -> (array with subset deleted=w377:string[])  [unwired: 1 out]
          n192 = Empty Array?(array=w377) -> (empty?=w379:bool)
          n193 = case shown="True" w379 {
            tunnel: [Aktionen_Zustandsfehlerinformation."OK" ("Aktionen") Aktionen_Zustandsfehlerinformation."Datenfehler" ("Aktionen")] -> w378
            tunnel: w377 -> [w387 _]
            tunnel: w376 -> [w386 _]
            tunnel: w375 -> [w385 _]
            tunnel: [w384 ""] -> w374
            frame False {
              # "Je nach Abgefragten Kanal den RICHTIGEN\nMesswert heraussuchen!"
              n194 = for {
                tunnel: w387 -> [w402] mode=indexing
                tunnel: w386 -> [w400]
                tunnel: w385 -> [w399]
                shift-right: [w398] -> w384
                shift-left: "" -> [w395]
                n195 = Decimal String To Number(string=w402, offset=1 ("Offset (0)")) -> (number=w394:i32)  [unwired: 1 in, 1 out]
                n196 = Decrement(x=w394) -> (x-1=w393:i32)
                n197 = Index Array(array=w400, index=w393) -> (element=w391:i16)
                n198 = Index Array(array=w399, index=w391) -> (element=w397:sgl)
                n199 = call <vilib>:"Space Constant.vi"() -> ("String"=w392:string)
                n200 = Number To Fractional String(use system decimal point (T)=FALSE ("Systemdezimalzeichen verwenden (T)"), number=w397, precision (6)=i16 2 ("Genauigkeit (6)")) -> (F-format string=w396:string)  [unwired: 1 in]
                n201 = Concatenate Strings(w395, w392, w396) -> (w398:string)
              }
            }
            frame True {
              # "Wenn der String leer ist, dann Datenfehler"
            }
          }
        }
        frame True {
          n202 = for {
            tunnel: w409 -> [w412] mode=indexing
            shift-right: [w418] -> w407
            shift-left: "" -> [w417]
            tunnel: w406 -> [w416]
            n203 = Index Array(array=w416, index=w412) -> (element=w415:sgl)
            n204 = Number To Fractional String(use system decimal point (T)=FALSE ("Systemdezimalzeichen verwenden (T)"), number=w415, precision (6)=i16 2 ("Genauigkeit (6)")) -> (F-format string=w414:string)  [unwired: 1 in]
            n205 = call <vilib>:"Space Constant.vi"() -> ("String"=w413:string)
            n206 = Concatenate Strings(w417, w413, w414) -> (w418:string)
          }
        }
      }
      n207 = call "Zustandsfehlerinformation.vi"("Aktionen"=w358, "String"=w365) -> ("String"=w364:string)  [unwired: 9 in]
      n208 = Concatenate Strings(w364, w361) -> (w366:string)
    }
    frame "AIKO" {
      # "Messwertabfrage"
      n209 = call "FGV Messdaten.vi"("Aktionen"=Aktionen_FGV_Messdaten."lesen") -> ("Aktuelle Messwerte"=w422:sgl[])  [unwired: 6 in, 8 out]
      n210 = call "FGV System.vi"("Aktionen"=Aktioen_FGV_System."lesen") -> ("Optionen"=w420:T20)  [unwired: 12 in, 6 out]
      n211 = Unbundle By Name(w420) -> ("AK in ppm"=w423:bool)
      n212 = call "Gespeicherte Werte.vi"("Aktionen"=Aktionen_Gespeicherte_Werte."lesen") -> ("Diverse Werte"=w431:T15)  [unwired: 6 in, 4 out]
      n213 = Index Array(array=w433, index=1 ("Index")) -> (element=w427:string)
      n214 = Unbundle By Name(w431) -> ("Gas-Reihenfolge"=w436:i16[])
      n215 = case shown="True" w423 {
        tunnel: w422 -> [w441 w443]
        tunnel: [w441 w442] -> w421
        frame False {
        }
        frame True {
          n216 = call "H2O und CO2 umrechnen.vi"("Aktuelle Messwerte"=w443) -> ("Aktuelle Messwerte"=w442:sgl[])  [unwired: 10 in]
        }
      }
      n217 = Equal?(x=w427, y="K0") -> (x = y?=w426:bool)
      n218 = Equal?(x=w427, y="KV") -> (x = y?=w425:bool)
      n219 = Or(x=w426, y=w425) -> (x .or. y?=w424:bool)
      n220 = case shown="True" w424 {
        tunnel: w436 -> [w446 w479]
        tunnel: [w444 w477] -> w435
        tunnel: w421 -> [w445 w476]
        tunnel: w433 -> [w450 _]
        tunnel: [w448 Aktionen_Zustandsfehlerinformation."OK" ("Aktionen")] -> w432
        frame False {
          n221 = Delete From Array(array=w450, length=1 ("Länge"), index=0 ("Index")) -> (array with subset deleted=w447:string[])  [unwired: 1 out]
          n222 = Empty Array?(array=w447) -> (empty?=w449:bool)
          n223 = case shown="False" w449 {
            tunnel: [Aktionen_Zustandsfehlerinformation."OK" ("Aktionen") Aktionen_Zustandsfehlerinformation."Datenfehler" ("Aktionen")] -> w448
            tunnel: w447 -> [w457 _]
            tunnel: w446 -> [w456 _]
            tunnel: w445 -> [w455 _]
            tunnel: [w454 ""] -> w444
            frame False {
              # "Je nach Abgefragten Kanal den RICHTIGEN\nMesswert heraussuchen!"
              n224 = for {
                tunnel: w457 -> [w472] mode=indexing
                tunnel: w456 -> [w470]
                tunnel: w455 -> [w469]
                shift-right: [w468] -> w454
                shift-left: "" -> [w465]
                n225 = Decimal String To Number(string=w472, offset=1 ("Offset (0)")) -> (number=w464:i32)  [unwired: 1 in, 1 out]
                n226 = Decrement(x=w464) -> (x-1=w463:i32)
                n227 = Index Array(array=w470, index=w463) -> (element=w461:i16)
                n228 = Index Array(array=w469, index=w461) -> (element=w467:sgl)
                n229 = call <vilib>:"Space Constant.vi"() -> ("String"=w462:string)
                n230 = Number To Fractional String(use system decimal point (T)=FALSE ("Systemdezimalzeichen verwenden (T)"), number=w467, precision (6)=i16 2 ("Genauigkeit (6)")) -> (F-format string=w466:string)  [unwired: 1 in]
                n231 = Concatenate Strings(w465, w462, w466) -> (w468:string)
              }
            }
            frame True {
              # "Wenn der String leer ist, dann Datenfehler"
            }
          }
        }
        frame True {
          n232 = for {
            tunnel: w479 -> [w482] mode=indexing
            shift-right: [w488] -> w477
            shift-left: "" -> [w487]
            tunnel: w476 -> [w486]
            n233 = Index Array(array=w486, index=w482) -> (element=w485:sgl)
            n234 = Number To Fractional String(use system decimal point (T)=FALSE ("Systemdezimalzeichen verwenden (T)"), number=w485, precision (6)=i16 2 ("Genauigkeit (6)")) -> (F-format string=w484:string)  [unwired: 1 in]
            n235 = call <vilib>:"Space Constant.vi"() -> ("String"=w483:string)
            n236 = Concatenate Strings(w487, w483, w484) -> (w488:string)
          }
        }
      }
      n237 = call "Zustandsfehlerinformation.vi"("Aktionen"=w432, "String"=w439) -> ("String"=w438:string)  [unwired: 9 in]
      n238 = Concatenate Strings(w438, w435) -> (w440:string)
    }
    frame "ASTF" {
      n239 = call "Zustandsfehlerinformation.vi"("Aktionen"=Aktionen_Zustandsfehlerinformation."OK", "String"=w493) -> ("String"=w492:string)  [unwired: 9 in]
      n240 = call "Fehler Zaehler.vi"("Aktionen"=Aktionen_Stoernummern_pruefen."lesen") -> ("Fehler Nummern"=w490:string)  [unwired: 7 in, 3 out]
      n241 = call <vilib>:"Space Constant.vi"() -> ("String"=w489:string)
      n242 = Concatenate Strings(w492, w489, w490) -> (w495:string)
    }
    frame "ASTZ" {
      n243 = Index Array(array=w510, index=1 ("Index")) -> (element=w503:string)
      n244 = call "Zustandsfehlerinformation.vi"("Aktionen"=Aktionen_Zustandsfehlerinformation."OK", "String"=w511) -> ("String"=w507:string)  [unwired: 9 in]
      n245 = call "FGV Schedule Status.vi"("Aktion"=Aktion_FGV_Scheduler_Status."lesen") -> ("Scheduler Status"=w496:bool)  [unwired: 13 in, 1 out]
      n246 = call "FGV-Funktionstasten.vi"("Aktion"=Funktionstasten-Aktion."Lesen") -> ("ausgewählte Funktion"=w499:T4, "Betriebsart"=w505:T5)  [unwired: 7 in, 6 out]
      n247 = case shown="True" w496 {
        tunnel: w499 -> [w513 _]
        tunnel: [w512 "SATK" ("String")] -> w498
        frame False {
          n248 = case shown="\"Init 4\"" w513 {
            tunnel: ["STBY" ("String") "SPAU" ("String") "SECO" ("String") "SMGA" ("String") "SATK" ("String") "SEKA" ("String") "SRUC" ("String") "SSPL" ("String") "SNGA" ("String") "SCZP" ("String") _ _ _ _ _ _ _ _] -> w512
            frame "Standby", Default {
            }
            frame "Pause" {
            }
            frame "Eco" {
            }
            frame "Messen" {
            }
            frame "Kalibrieren" {
            }
            frame "Cal-Gas" {
              # "#KaliAutoMessenBug"
            }
            frame "Spülen Filter" {
            }
            frame "Spülen Leitung" {
            }
            frame "0-Gas" {
            }
            frame "CG zu PNS" {
              # "#KaliAutoMessenBug"
            }
            frame "Init 1" {
            }
            frame "Init 2" {
            }
            frame "-------------" {
            }
            frame "Init 3" {
            }
            frame "Init 4" {
            }
            frame "Messen vorbereiten" {
            }
            frame "Messen durchführen" {
            }
            frame "Exit" {
            }
          }
        }
        frame True {
        }
      }
      n249 = case shown="\"KV\"" w503 {
        selector: w503 -> [w525 _ _]
        tunnel: [w525 "K1" ("String") "KV" ("String")] -> w502
        frame "K1", Default {
        }
        frame "K0" {
        }
        frame "KV" {
        }
      }
      n250 = case shown="\"Manuell\", Standard" w505 {
        tunnel: ["SMAN" ("String") "SREM" ("String") "SBIT" ("String")] -> w501
        frame "Manuell", Default {
        }
        frame "Remote" {
        }
        frame "Bitparallel" {
        }
      }
      n251 = call <vilib>:"Space Constant.vi"() -> ("String"=w500:string)
      n252 = Concatenate Strings(w507, w500, w502, w500, w501, w500, w498) -> (w509:string)
      n253 = disable-structure shown="Deaktiviert" {
        frame Disabled {
          n254 = Index Array(index=1 ("Index")) -> (element=w532)  [unwired: 1 in]
          n255 = call "Zustandsfehlerinformation.vi"("Aktionen"=Aktionen_Zustandsfehlerinformation."OK") -> (2:"String"=w535:string, 10:"String"=w537:string)  [unwired: 9 in]
          n256 = call "ASTZ - AVL Sesam.vi"("Selektor"=w532) -> ("Verknüpfter String"=w531:string)  [unwired: 10 in]
          n257 = call <vilib>:"Space Constant.vi"() -> ("String"=w533:string)
          n258 = Concatenate Strings(w535, w533, w531) -> ()  [unwired: 1 out]
        }
        frame Enabled {
        }
      }
    }
    frame "ATEM" {
      n259 = call "FGV cRIO-Daten.vi"("Aktion"=enum16{"lesen", "schreiben"}."lesen") -> ("TC Eingänge"=w538:T21)  [unwired: 9 in, 9 out]
      n260 = call "Zustandsfehlerinformation.vi"("Aktionen"=Aktionen_Zustandsfehlerinformation."OK", "String"=w563) -> ("String"=w562:string)  [unwired: 9 in]
      n261 = Unbundle By Name(w538) -> ("TC1: HL zu FT-IR"=w545:sgl, "TC2: HL Extern SP1"=w544:sgl, "TC3: HL Extern SP2"=w541:sgl, "TC4: Reserve"=w543:sgl)
      n262 = call "FGV FT-IR Diagnosewerte.vi"("Aktionen"=FGV_FT-IR_Diagnose_Aktionen."Lesen") -> ("Temperatur"=w556:dbl)  [unwired: 5 in, 5 out]
      n263 = Number To Fractional String(use system decimal point (T)=FALSE ("Systemdezimalzeichen verwenden (T)"), number=w556, precision (6)=i16 1 ("Genauigkeit (6)")) -> (F-format string=w559:string)  [unwired: 1 in]
      n264 = Number To Fractional String(use system decimal point (T)=FALSE ("Systemdezimalzeichen verwenden (T)"), number=w545, precision (6)=i16 1 ("Genauigkeit (6)")) -> (F-format string=w553:string)  [unwired: 1 in]
      n265 = Number To Fractional String(use system decimal point (T)=FALSE ("Systemdezimalzeichen verwenden (T)"), number=w544, precision (6)=i16 1 ("Genauigkeit (6)")) -> (F-format string=w550:string)  [unwired: 1 in]
      n266 = Number To Fractional String(use system decimal point (T)=FALSE ("Systemdezimalzeichen verwenden (T)"), number=w541, precision (6)=i16 1 ("Genauigkeit (6)")) -> (F-format string=w542:string)  [unwired: 1 in]
      n267 = Number To Fractional String(use system decimal point (T)=FALSE ("Systemdezimalzeichen verwenden (T)"), number=w543, precision (6)=i16 1 ("Genauigkeit (6)")) -> (F-format string=w540:string)  [unwired: 1 in]
      n268 = call <vilib>:"Space Constant.vi"() -> ("String"=w539:string)
      n269 = Concatenate Strings(w562, w539, w559, w539, w553, w539, w550, w539, w542, w539, w540) -> (w565:string)
    }
    frame "EFDA" {
      n270 = Index Array(array=w570, index #1=2 ("Index"), index #2=3 ("Index")) -> (element #1=w567:string, element #2=w566:string)
      n271 = case shown="\"SNGA\"" w567 {
        tunnel: w572 -> [w574 w585 w595]
        tunnel: [w573 w584 w594] -> w571
        tunnel: w566 -> [_ w577 w587]
        frame " ", Default {
          n272 = call "Zustandsfehlerinformation.vi"("Aktionen"=Aktionen_Zustandsfehlerinformation."Datenfehler", "String"=w574) -> ("String"=w573:string)  [unwired: 9 in]
        }
        frame "SNGA" {
          n273 = Decimal String To Number(string=w577, default (0L)=sgl 0.0) -> (number=w576:sgl)  [unwired: 1 in, 1 out]
          n274 = call "Zustandsfehlerinformation.vi"("Aktionen"=Aktionen_Zustandsfehlerinformation."OK", "String"=w585) -> ("String"=w584:string)  [unwired: 9 in]
          n275 = call "Gespeicherte Werte.vi"("Aktionen"=Aktionen_Gespeicherte_Werte."lesen") -> ("Diverse Werte"=w580:T15)  [unwired: 6 in, 4 out]
          n276 = Bundle By Name(cluster=w580, "Zeit 0-Gas"=w576) -> (w579:T15)
          n277 = call "Gespeicherte Werte.vi"("Aktionen"=Aktionen_Gespeicherte_Werte."Diverse", "Diverse Werte"=w579) -> ()  [unwired: 5 in, 5 out]
        }
        frame "SEGA" {
          n278 = Decimal String To Number(string=w587, default (0L)=sgl 0.0) -> (number=w586:sgl)  [unwired: 1 in, 1 out]
          n279 = call "Zustandsfehlerinformation.vi"("Aktionen"=Aktionen_Zustandsfehlerinformation."OK", "String"=w595) -> ("String"=w594:string)  [unwired: 9 in]
          n280 = call "Gespeicherte Werte.vi"("Aktionen"=Aktionen_Gespeicherte_Werte."lesen") -> ("Diverse Werte"=w590:T15)  [unwired: 6 in, 4 out]
          n281 = Bundle By Name(cluster=w590, "Zeit CalGas"=w586) -> (w589:T15)
          n282 = call "Gespeicherte Werte.vi"("Aktionen"=Aktionen_Gespeicherte_Werte."Diverse", "Diverse Werte"=w589) -> ()  [unwired: 5 in, 5 out]
        }
      }
    }
    frame "EKFG" {
      n283 = Index Array(array=w601, index=1 ("Index")) -> (element=w596:string)
      n284 = case shown="\"K1\"" w596 {
        tunnel: w601 -> [_ w606 w632]
        tunnel: [Aktionen_Zustandsfehlerinformation."Syntax Error" ("Aktionen") w603 w629] -> w597
        frame " ", Default {
          # "Befehlskomando NICHT KORREKT!"
        }
        frame "K1" {
          n285 = Delete From Array(array=w606, length=2 ("Länge"), index=0 ("Index")) -> (array with subset deleted=w605:string[])  [unwired: 1 out]
          n286 = Empty Array?(array=w605) -> (empty?=w604:bool)
          n287 = case shown="False" w604 {
            tunnel: w605 -> [w615 _]
            tunnel: [w612 Aktionen_Zustandsfehlerinformation."Datenfehler" ("Aktionen")] -> w603
            frame False {
              n288 = call "Gespeicherte Werte.vi"("Aktionen"=Aktionen_Gespeicherte_Werte."lesen") -> ()  [unwired: 6 in, 5 out]
              n289 = call "AK Namen.vi"("Aktionen"=AK_Namen_Aktionen."lesen") -> ("AK Namen"=w609:string[])  [unwired: 7 in, 3 out]
              n290 = for {
                tunnel: w615 -> [w618] mode=indexing
                tunnel: [w617] -> w614 mode=indexing
                tunnel: w609 -> [w619]
                tunnel: [w620] -> w611
                stop <- w620 stop-if-true
                n291 = call "String suchen AK.vi"("gesucht"=w618, "Namen"=w619) -> ("Index"=w617:i32, "Gefunden?"=w616:bool)  [unwired: 8 in]
                n292 = Not(x=w616) -> (.not. x?=w620:bool)
              }
              n293 = case shown="False" w611 {
                tunnel: w614 -> [w625 _]
                tunnel: [Aktionen_Zustandsfehlerinformation."OK" ("Aktionen") Aktionen_Zustandsfehlerinformation."Datenfehler" ("Aktionen")] -> w612
                frame False {
                  n294 = call "Gespeicherte Werte.vi"("Aktionen"=Aktionen_Gespeicherte_Werte."lesen") -> ("Diverse Werte"=w623:T15)  [unwired: 6 in, 4 out]
                  n295 = Bundle By Name(cluster=w623, "Gas-Reihenfolge"=w625) -> (w622:T15)
                  n296 = call "Gespeicherte Werte.vi"("Aktionen"=Aktionen_Gespeicherte_Werte."Diverse", "Diverse Werte"=w622) -> ()  [unwired: 5 in, 5 out]
                }
                frame True {
                }
              }
            }
            frame True {
              # "Fehler mit den Einstell Kommandos"
            }
          }
        }
        frame "KV" {
          n297 = Delete From Array(array=w632, length=3 ("Länge"), index=0 ("Index")) -> (array with subset deleted=w631:string[])  [unwired: 1 out]
          n298 = Empty Array?(array=w631) -> (empty?=w630:bool)
          n299 = case shown="False" w630 {
            tunnel: w631 -> [w638 _]
            tunnel: [w637 Aktionen_Zustandsfehlerinformation."Datenfehler" ("Aktionen")] -> w629
            frame False {
              n300 = for {
                tunnel: w638 -> [w640] mode=indexing
                tunnel: [w639] -> w636 mode=indexing
                n301 = Decimal String To Number(string=w640, offset=1 ("Offset")) -> (number=w639:i32)  [unwired: 1 in, 1 out]
              }
              n302 = Empty Array?(array=w636) -> (empty?=w635:bool)
              n303 = case shown="False" w635 {
                tunnel: w636 -> [w646 _]
                tunnel: [Aktionen_Zustandsfehlerinformation."OK" ("Aktionen") Aktionen_Zustandsfehlerinformation."Datenfehler" ("Aktionen")] -> w637
                frame False {
                  n304 = call "Gespeicherte Werte.vi"("Aktionen"=Aktionen_Gespeicherte_Werte."lesen") -> ("Diverse Werte"=w644:T15)  [unwired: 6 in, 4 out]
                  n305 = Bundle By Name(cluster=w644, "Gas-Reihenfolge"=w646) -> (w643:T15)
                  n306 = call "Gespeicherte Werte.vi"("Aktionen"=Aktionen_Gespeicherte_Werte."Diverse", "Diverse Werte"=w643) -> ()  [unwired: 5 in, 5 out]
                }
                frame True {
                }
              }
            }
            frame True {
              # "Fehler mit den Einstell Kommandos"
            }
          }
        }
      }
      n307 = call "Zustandsfehlerinformation.vi"("Aktionen"=w597, "String"=w600) -> ("String"=w599:string)  [unwired: 9 in]
    }
  }
  "String für schreiben" <- w5
